vi "createADCScanRateFrame.vi"(8 "error in (no error)":errorcluster, 9 "TriggerIRQ":bool, 10 "WaitForTrigger":bool, 11 "ILC in":refnum<class "ILC.lvclass">) -> (0 "error out":errorcluster, 2 "TxFrame":T1 {"Data" format="%02x"}, 3 "ILC out":refnum<class "ILC.lvclass">)   [LabVIEW 2016, in "RTILC.lvlib" / "ILC.lvclass"]
uses:
  ILC.lvclass
  Common_RT_Modbus/DataTypes/TxFrame.ctl
  Common_RT_Modbus/DynamicFrameBuilder/DynamicFrameBuilder.lvclass
  Common_RT_Modbus/DataTypes/ExceptionCodes.ctl
  ILC.lvclass/ILC.ctl
  Common_RT_Modbus/RTModbus.lvlib
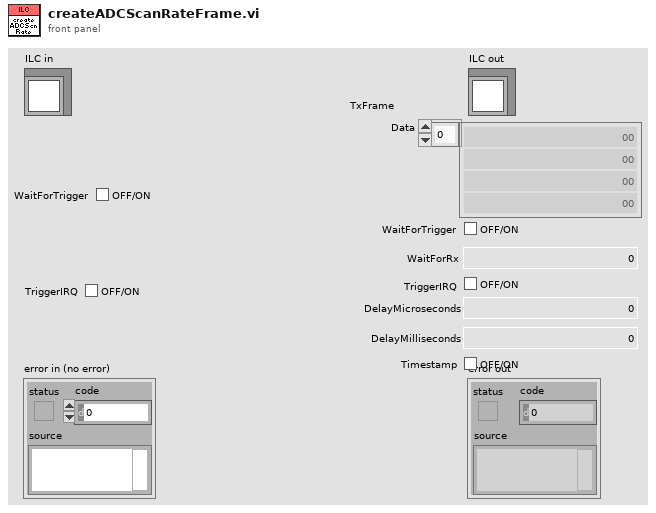
[diagram p1: front panel]
types:
  T1 = typedef "RTModbus.lvlib/TxFrame.ctl" = cluster{"Data":u8[], "WaitForTrigger":bool, "WaitForRx":u32, "TriggerIRQ":bool, "DelayMicroseconds":u16, "DelayMilliseconds":u16, "Timestamp":bool}
  T2 = typedef "RTModbus.lvlib/ExceptionCodes.ctl" = u16
  T3 = typedef "RTILC.lvlib/ILCScanRates.ctl" = u8
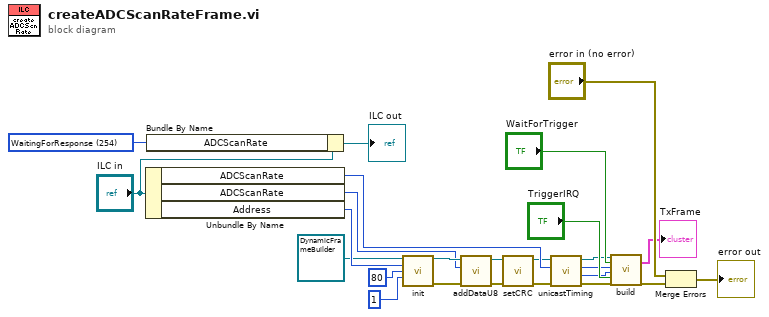
[diagram p0: block diagram]
diagram:
  w3 = T2 254 items=["OK"=0, "IllegalFunction"=1, "IllegalDataAddress"=2, "IllegalDataValue"=3, "SlaveDeviceFailure"=4, "Acknowledge"=5, "SlaveDeviceBusy"=6, "NegativeAcknowledge"=7, "MemoryParityError"=8, "GatewayPathUnavailable"=9, "GatewayTargetDeviceFailedToRespond"=10, "WaitingForResponse"=254, "CRCError"=255] ("ILCData.Responses.ADCOffsetSensitivity")
  n1 = Unbundle By Name("ILC in") -> ("ADCScanRate"=w10:u32, "ADCScanRate"=w18:T3, "Address"=w21:u8)
  n2 = Bundle By Name(cluster="ILC in", "ADCScanRate"=w3) -> (→"ILC out":refnum<class "ILC.lvclass">)
  n3 = call "init.vi"("DynamicFrameBuilder in"=refnum<class "DynamicFrameBuilder.lvclass"> refnum ("RTModbus.lvlib:DynamicFrameBuilder.lvclass"), "Address"=w21, "Function"=u8 80, "DataSize"=1) -> ("DynamicFrameBuilder out"=w19:refnum<class "DynamicFrameBuilder.lvclass">, "error out"=w17:errorcluster)  [unwired: 10 in]
  n4 = call "addDataU8.vi"("error in (no error)"=w17, "Data"=w18, "DynamicFrameBuilder in"=w19) -> ("error out"=w15:errorcluster, "DynamicFrameBuilder out"=w16:refnum<class "DynamicFrameBuilder.lvclass">)  [unwired: 7 in]
  n5 = call "setCRC.vi"("error in (no error)"=w15, "DynamicFrameBuilder in"=w16) -> ("error out"=w8:errorcluster, "DynamicFrameBuilder out"=w9:refnum<class "DynamicFrameBuilder.lvclass">)  [unwired: 8 in]
  n6 = call "unicastTiming.vi"("error in (no error)"=w8, "Latency in"=w10, "DynamicFrameBuilder in"=w9) -> ("error out"=w7:errorcluster, "WaitForRxTimeout"=w4:u32, "Latency out"=w5:u32, "DynamicFrameBuilder out"=w6:refnum<class "DynamicFrameBuilder.lvclass">)  [unwired: 5 in]
  n7 = call "build.vi"("DynamicFrameBuilder in"=w6, "WaitForTrigger"="WaitForTrigger", "Latency"=w5, "WaitForRxTimeout"=w4, "TriggerIRQ"="TriggerIRQ", "error in (no error)"=w7) -> ("TxFrame"=→"TxFrame":T1, "error out"=w11:errorcluster)  [unwired: 11 in, 1 out]
  n8 = Merge Errors("error in (no error)", w11) -> (→"error out":errorcluster)
